vi "Set Ramp Rate Units.vi"(8 "error in":T2, 9 "Ramp Rate Units":u16(ring) items=["Per SECOND", "Per MINUTE"], 11 "Communications Config":T1={"connection ID"=refnum, "IP"="192.168.0.108", "Active Comm Interface"=0, "Serial Port"="", "Programmer Type"=0, "connection ID"=refnum, "output cluster"={"GPIB address"=0, "GPIB bus"=0}} {"Programmer Type" items=["Model 430", "Model 420"]; "Active Comm Interface" items=["TCP/IP (Model 430 Only)", "RS232", "IEEE488"]}) -> (0 "error out":T2)   [LabVIEW 2017]
uses:
  commsControl.ctl
panel:
  in  "GPIB Address":cluster{"GPIB address":i16, "GPIB bus":i16}={"GPIB address"=22, "GPIB bus"=0}
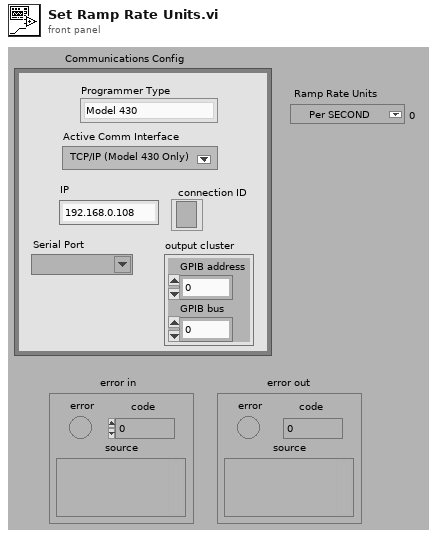
[diagram p1: front panel]
types:
  T1 = typedef "commsControl.ctl" = cluster{"connection ID":refnum<k5>, "IP":string, "Active Comm Interface":u16, "Serial Port":refnum<visa-resource-name>, "Programmer Type":u16, "connection ID":refnum<k5>, "output cluster":cluster{"GPIB address":i16, "GPIB bus":i16}}
  T2 = cluster{"error":bool, "code":i32, "source":string}
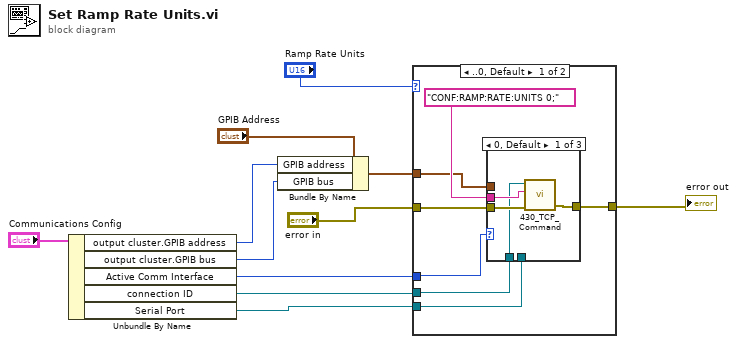
[diagram p0: block diagram]
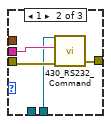
[diagram p2: hidden frame]
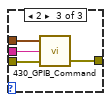
[diagram p3: hidden frame]
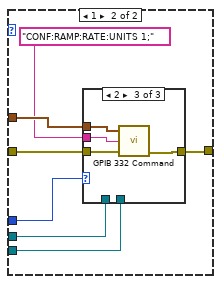
[diagram p4: hidden frame]
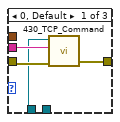
[diagram p5: hidden frame]
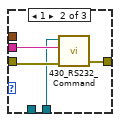
[diagram p6: hidden frame]
diagram:
  n1 = Unbundle By Name("Communications Config") -> ("output cluster.GPIB address"=w7:i16, "output cluster.GPIB bus"=w6:i16, "Active Comm Interface"=w4:u16, "connection ID"=w3:refnum<k5>, "Serial Port"=w2:refnum<visa-resource-name>)
  n2 = Bundle By Name(cluster="GPIB Address", "GPIB address"=w7, "GPIB bus"=w6) -> (w5:cluster{"GPIB address":i16, "GPIB bus":i16})
  n3 = case shown="..0, Default" "Ramp Rate Units" {
    tunnel: w5 -> [w14 w37]
    tunnel: "error in" -> [w17 w35]
    tunnel: [w16 w34] -> w9
    tunnel: w4 -> [w15 w33]
    tunnel: w3 -> [w13 w32]
    tunnel: w2 -> [w12 w31]
    frame ..0, Default {
      n4 = case shown="0, Default" w15 {
        tunnel: w14 -> [_ _ w30]
        tunnel: "CONF:RAMP:RATE:UNITS 0;" -> [w20 w24 w29]
        tunnel: w17 -> [w21 w25 w28]
        tunnel: [w22 w26 w27] -> w16
        tunnel: w13 -> [w19 _ _]
        tunnel: w12 -> [_ w23 _]
        frame 0, Default {
          n5 = call "430_TCP_Command.vi"("error in (no error)"=w21, "Command"=w20, "connection ID"=w19) -> ("error out"=w22:errorcluster)  [unwired: 1 in, 2 out]
        }
        frame 1 {
          n6 = call "430_RS232_Command.vi"("error in (no error)"=w25, "Command"=w24, "VISA resource name"=w23) -> ("error out"=w26:errorcluster)  [unwired: 1 in, 2 out]
        }
        frame 2 {
          n7 = call "430_GPIB_Command.vi"("GPIB (In)"=w30, "Input command"=w29, "error in"=w28) -> ("error out"=w27:T2)  [unwired: 3 out]
        }
      }
    }
    frame 1 {
      n8 = case shown="2" w33 {
        tunnel: w37 -> [_ _ w49]
        tunnel: "CONF:RAMP:RATE:UNITS 1;" -> [w39 w43 w48]
        tunnel: w35 -> [w40 w44 w47]
        tunnel: [w41 w45 w46] -> w34
        tunnel: w32 -> [w38 _ _]
        tunnel: w31 -> [_ w42 _]
        frame 0, Default {
          n9 = call "430_TCP_Command.vi"("error in (no error)"=w40, "Command"=w39, "connection ID"=w38) -> ("error out"=w41:errorcluster)  [unwired: 1 in, 2 out]
        }
        frame 1 {
          n10 = call "430_RS232_Command.vi"("error in (no error)"=w44, "Command"=w43, "VISA resource name"=w42) -> ("error out"=w45:errorcluster)  [unwired: 1 in, 2 out]
        }
        frame 2 {
          n11 = call "GPIB 332 Command.vi"("GPIB (In)"=w49, "Input command"=w48, "error in"=w47) -> ("error out"=w46:T2)  [unwired: 3 out]
        }
      }
    }
  }
  "error out" <- w9
